vi "Write Allow.vi"(8 "error in (no error)":errorcluster, 10 "Allow":refnum<class "Interlock.lvclass">[](array[class]), 11 "Interlock Chain in":refnum<class "Interlock Chain.lvclass">) -> (0 "error out":errorcluster, 3 "Interlock Chain out":refnum<class "Interlock Chain.lvclass">)   [LabVIEW 2015, in "Interlocks.lvlib" / "Interlock Chain.lvclass"]
uses:
  Interlock Chain.lvclass
  Interlock/Interlock.lvclass
  Interlock Chain.lvclass/Interlock Chain.ctl
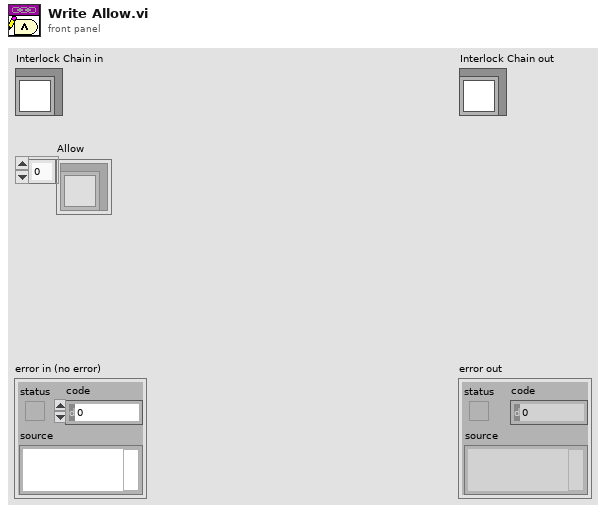
[diagram p1: front panel]
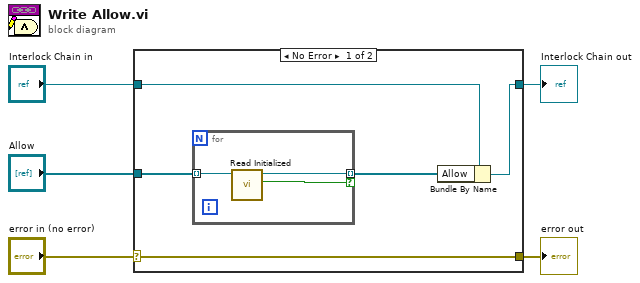
[diagram p0: block diagram]
diagram:
  n1 = case shown="No Error" "error in (no error)" {
    selector: "error in (no error)" -> [w10 w14]
    tunnel: [w10 w14] -> w4
    tunnel: [w8 w15] -> w2
    tunnel: "Interlock Chain in" -> [w9 w15]
    tunnel: "Allow" -> [w7 _]
    frame No Error {
      n2 = for {
        tunnel: w7 -> [w13] mode=indexing
        tunnel: [w12] -> w6 mode=indexing if=w11
        n3 = call-dynamic "Read Initialized.vi"("Interlock in"=w13) -> ("Initialized"=w11:bool, "Interlock out"=w12:refnum<class "Interlock.lvclass">)  [unwired: 9 in]
      }
      n4 = Bundle By Name(cluster=w9, "Allow"=w6) -> (w8:refnum<class "Interlock Chain.lvclass">)
    }
    frame Error {
    }
  }
  "error out" <- w4
  "Interlock Chain out" <- w2
